vi "WindowPositions.vi"(4 "Komunikat":refnum<vi>, 6 "WindowHandler":refnum<vi>, 7 "Dim":T1={"Width"=300, "Height"=170}, 8 "error in (no error)":errorcluster, 9 "Stop":refnum<vi>, 10 "Tab":refnum<vi>, 11 "VI in":refnum<vi>) -> (0 "error out":errorcluster)   [LabVIEW 2021]
uses:
  <vilib>/Utility/miscctls.llb/LVBoundsTypeDef.ctl
  <vilib>/Utility/miscctls.llb/LVRectTypeDef.ctl
  <vilib>/Utility/miscctls.llb/LVPointTypeDef.ctl
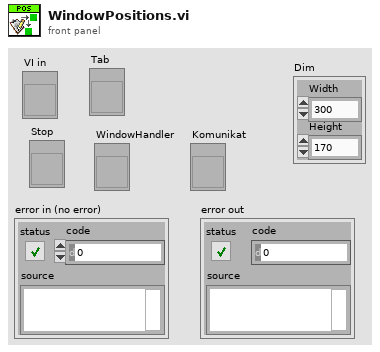
[diagram p1: front panel]
types:
  T1 = typedef "LVBoundsTypeDef.ctl" = cluster{"Width":u32, "Height":u32}
  T2 = typedef "LVPointTypeDef.ctl" = cluster{"Horizontal":i16, "Vertical":i16}
  T3 = typedef "LVRectTypeDef.ctl" = cluster{"Left":i16, "Top":i16, "Right":i16, "Bottom":i16}
  T4 = cluster{"Left":dbl, "Top":dbl, "Right":dbl, "Bottom":dbl}
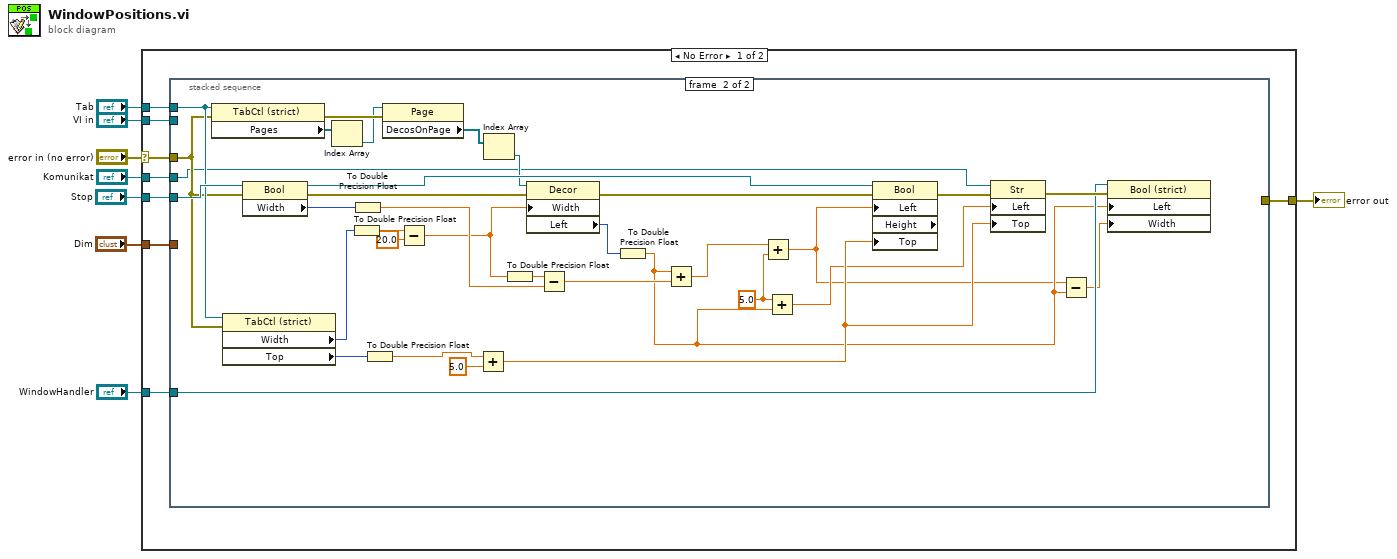
[diagram p0: block diagram]
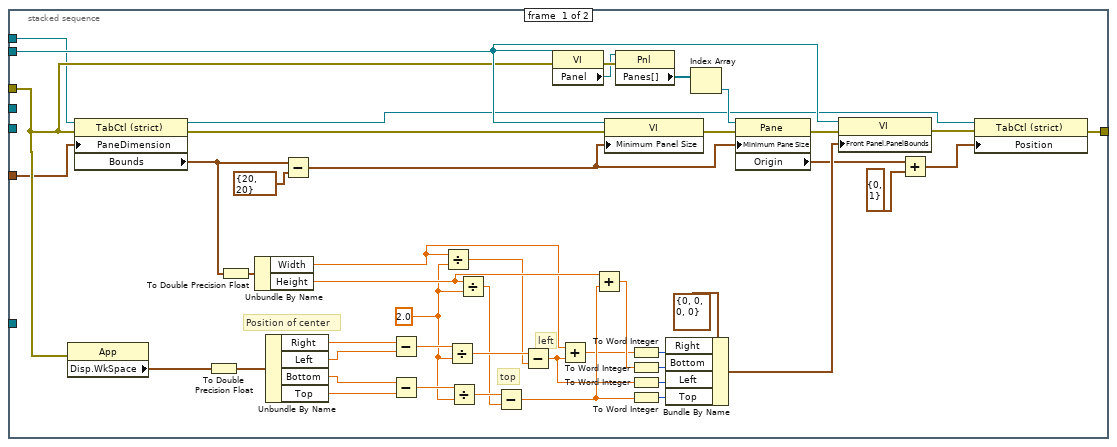
[diagram p2: hidden frame]
diagram:
  n1 = case shown="No Error" "error in (no error)" {
    selector: "error in (no error)" -> [w13 w97]
    tunnel: [w16 w97] -> w8
    tunnel: "Tab" -> [w15 _]
    tunnel: "VI in" -> [w14 _]
    tunnel: "Stop" -> [w12 _]
    tunnel: "Komunikat" -> [w11 _]
    tunnel: "WindowHandler" -> [w10 _]
    tunnel: "Dim" -> [w9 _]
    frame No Error {
      n2 = stacked-sequence {
        tunnel: [w62 _] -> w16
        tunnel: w15 -> [w20 w87]
        tunnel: w14 -> [w30 _]
        tunnel: w13 -> [w23 w86]
        tunnel: w12 -> [_ w88]
        tunnel: w11 -> [_ w85]
        tunnel: w10 -> [_ w69]
        tunnel: w9 -> [w17 _]
        frame #0 {
          w37 = 2.0
          # "Position of center"
          # "left"
          # "top"
          n3 = property class="App"(error in=w23) -> ("Disp.WkSpace"=w24:T3)  [unwired: 1 in, 2 out]
          n4 = property class="TabCtl (strict)"(reference=w20, error in=w23, "PaneDimension"=w17) -> (reference out=w22:refnum<vi>, error out=w21:errorcluster, "Bounds"=w18:T1)
          n5 = To Double Precision Float(number=w24) -> (double precision float=w48:T4)
          n6 = To Double Precision Float(number=w18) -> (double precision float=w54:cluster{"Width":dbl, "Height":dbl})
          n7 = Unbundle By Name(w54) -> ("Width"=w36:dbl, "Height"=w56:dbl)
          n8 = Unbundle By Name(w48) -> ("Right"=w44:dbl, "Left"=w45:dbl, "Bottom"=w46:dbl, "Top"=w47:dbl)
          n9 = Subtract(x=w18, y=T2 {"Horizontal"=20, "Vertical"=20} ("Minimum Pane Size")) -> (x-y=w61:T1)
          n10 = Subtract(x=w44, y=w45) -> (x-y=w49:dbl)
          n11 = Subtract(x=w46, y=w47) -> (x-y=w50:dbl)
          n12 = Divide(x=w36, y=w37) -> (x/y=w35:dbl)
          n13 = Divide(x=w49, y=w37) -> (x/y=w38:dbl)
          n14 = Divide(x=w50, y=w37) -> (x/y=w39:dbl)
          n15 = Divide(x=w56, y=w37) -> (x/y=w34:dbl)
          n16 = Subtract(x=w39, y=w34) -> (x-y=w43:dbl)
          n17 = Subtract(x=w38, y=w35) -> (x-y=w42:dbl)
          n18 = property class="VI"(reference=w30, error in=w23) -> (error out=w59:errorcluster, "Panel"=w57:refnum<vi>)  [unwired: 1 out]
          n19 = Add(x=w36, y=w42) -> (x+y=w40:dbl)
          n20 = Add(x=w56, y=w43) -> (x+y=w41:dbl)
          n21 = property class="VI"(reference=w30, error in=w21, "Minimum Panel Size"=w61) -> (error out=w32:errorcluster)  [unwired: 1 out]
          n22 = property class="Pnl"(reference=w57, error in=w59) -> ("Panes[]"=w58:refnum<vi>[])  [unwired: 2 out]
          n23 = To Word Integer(number=w40) -> (16bit integer=w51:i16)
          n24 = To Word Integer(number=w41) -> (16bit integer=w53:i16)
          n25 = To Word Integer(number=w42) -> (16bit integer=w52:i16)
          n26 = To Word Integer(number=w43) -> (16bit integer=w55:i16)
          n27 = Bundle By Name(cluster=T3 {"Left"=0, "Top"=0, "Right"=0, "Bottom"=0} ("Front Panel Window:Panel Bounds"), "Right"=w51, "Bottom"=w53, "Left"=w52, "Top"=w55) -> (w29:T3)
          n28 = Index Array(array=w58) -> (element=w60:refnum<vi>)  [unwired: 1 in]
          n29 = property class="Pane"(reference=w60, error in=w32, "Minimum Pane Size"=w61) -> (error out=w31:errorcluster, "Origin"=w28:T2)  [unwired: 1 out]
          n30 = property class="VI"(reference=w30, error in=w31, "Front Panel.PanelBounds"=w29) -> (error out=w26:errorcluster)  [unwired: 1 out]
          n31 = Add(x=w28, y=T2 {"Horizontal"=0, "Vertical"=1}) -> (x+y=w27:T2)
          n32 = property class="TabCtl (strict)"(reference=w22, error in=w26, "Position"=w27) -> (error out=w62:errorcluster)  [unwired: 1 out]
        }
        frame #1 {
          w65 = 5.0 ("y")
          n33 = property class="TabCtl (strict)"(reference=w87, error in=w86) -> (error out=w92:errorcluster, "Pages"=w91:refnum<vi>[])  [unwired: 1 out]
          n34 = property class="TabCtl (strict)"(reference=w87, error in=w86) -> ("Width"=w75:u32, "Top"=w76:i32)  [unwired: 2 out]
          n35 = property class="Bool"(reference=w88, error in=w86) -> (reference out=w95:refnum<vi>, error out=w96:errorcluster, "Width"=w81:u32)
          n36 = Index Array(array=w91) -> (element=w90:refnum<vi>)  [unwired: 1 in]
          n37 = To Double Precision Float(number=w75) -> (double precision float=w74:dbl)
          n38 = To Double Precision Float(number=w81) -> (double precision float=w80:dbl)
          n39 = To Double Precision Float(number=w76) -> (double precision float=w77:dbl)
          n40 = property on="Property Node" class="Page"(reference=w90, error in=w92) -> ("DecosOnPage"=w93:refnum<vi>[])  [unwired: 2 out]
          n41 = Subtract(x=w74, y=20.0) -> (x-y=w72:dbl)
          n42 = Add(x=w77, y=5.0) -> (x+y=w83:dbl)
          n43 = Index Array(array=w93) -> (element=w89:refnum<vi>)  [unwired: 1 in]
          n44 = To Double Precision Float(number=w72) -> (double precision float=w79:dbl)
          n45 = property class="Decor"(reference=w89, error in=w96, "Width"=w72) -> (error out=w94:errorcluster, "Left"=w78:i32)  [unwired: 1 out]
          n46 = Subtract(x=w79, y=w80) -> (x-y=w71:dbl)
          n47 = To Double Precision Float(number=w78) -> (double precision float=w66:dbl)
          n48 = Add(x=w66, y=w71) -> (x+y=w64:dbl)
          n49 = Add(x=w64, y=w65) -> (x+y=w63:dbl)
          n50 = Add(x=w65, y=w66) -> (x+y=w67:dbl)
          n51 = property class="Bool" props=["Left", "Height", "Top"](reference=w95, error in=w94, "Left"=w63, "Top"=w83) -> (error out=w84:errorcluster)  [unwired: 2 out]
          n52 = property class="Str"(reference=w85, error in=w84, "Left"=w67, "Top"=w83) -> (error out=w70:errorcluster)  [unwired: 1 out]
          n53 = Subtract(x=w63, y=w66) -> (x-y=w68:dbl)
          n54 = property class="Bool (strict)"(reference=w69, error in=w70, "Left"=w66, "Width"=w68) -> ()  [unwired: 2 out]
        }
      }
    }
    frame Error {
    }
  }
  "error out" <- w8
